vi "Replace Array Elements.vi"() -> ()   [LabVIEW 2019]
doc: "Demonstrates the use of the Replace Array Subset function."
panel:
  out "Case 4 - Replace One Column in 2D Array":dbl[][](array[numeric])
  out "Case 3 - Replace One Row in 2D Array":dbl[][](array[numeric])
  in  "Column Index":i32
  in  "Row Index":i32
  in  "Element Index":i32
  in  "New Element":dbl=9.99
  out "Case 2 - Replace One Element in 2D Array":dbl[][](array[numeric])
  out "Case 1 - Replace One Element in 1D Array":dbl[](array[numeric])
  in  "Original 2D Array":dbl[][](array[numeric])=[[0.0, 1.0, 2.0, 3.0], [4.0, 5.0, 6.0, 7.0], [8.0, 9.0, 10.0, 11.0], [12.0, 13.0, 14.0, 15.0]]
  in  "Original 1D Array":dbl[](array[numeric])=[100.0, 101.0, 102.0, 103.0]
  # "Overview: Demonstrates the use of the Replace Array Subset function.\nInstructions:\nRun the VI."
  # "Assign New Element into the 1D array at the position specified by Element Index."
  # "Assign New Element into the 2D array at the position specified by Row Index and Column Index."
  # "Assign Original 1D Array into the 2D array at the row specified by Row Index."
  # "Assign Original 1D Array into the 2D array at the column specified by Column Index."
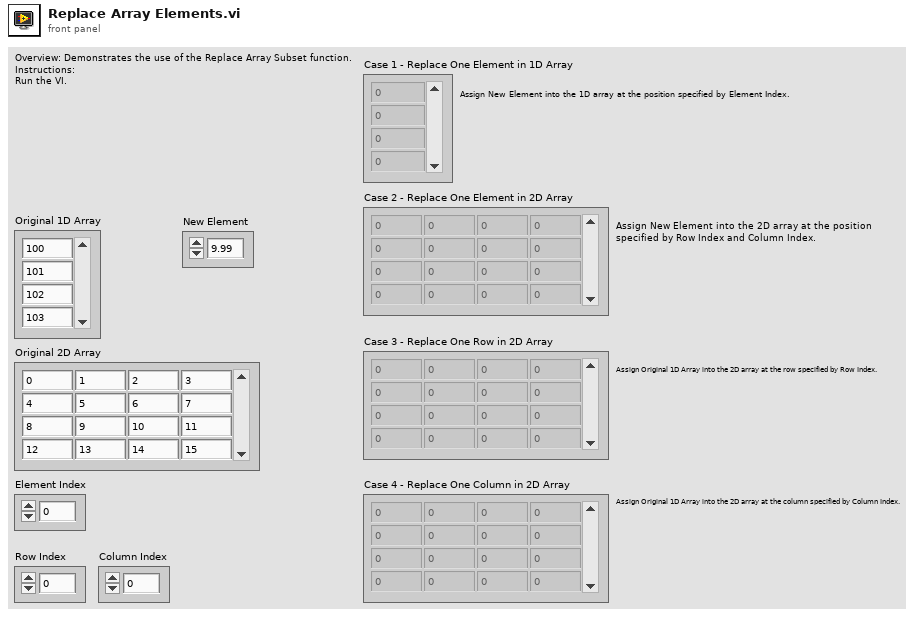
[diagram p1: front panel]
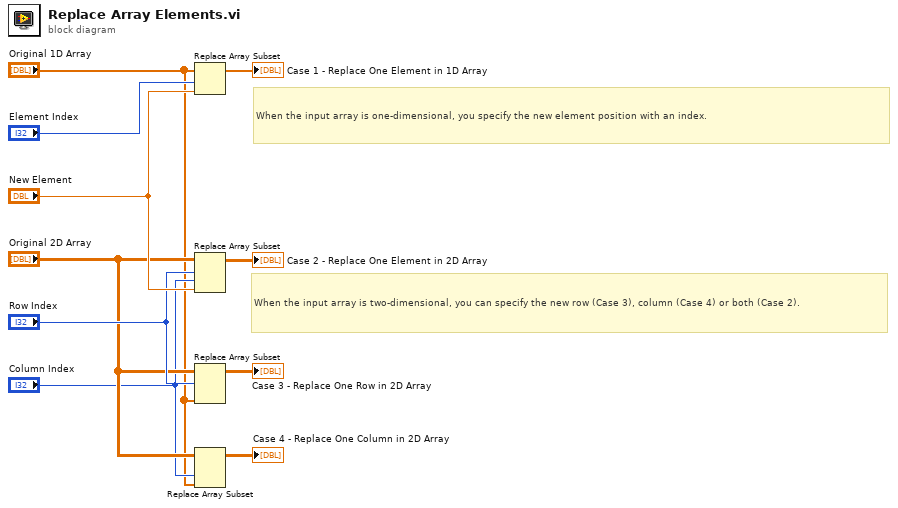
[diagram p0: block diagram]
diagram:
  # "When the input array is two-dimensional, you can specify the new row (Case 3), column (Case 4) or both (Case 2)."
  # "When the input array is one-dimensional, you specify the new element position with an index."
  n1 = Replace Array Subset(array="Original 1D Array", new element="New Element", index="Element Index") -> (→"Case 1 - Replace One Element in 1D Array":dbl[])
  n2 = Replace Array Subset(array="Original 2D Array", new element="New Element", index (row)="Row Index", index (col)="Column Index") -> (→"Case 2 - Replace One Element in 2D Array":dbl[][])
  n3 = Replace Array Subset(array="Original 2D Array", new element="Original 1D Array", index (row)="Row Index") -> (→"Case 3 - Replace One Row in 2D Array":dbl[][])  [unwired: 1 in]
  n4 = Replace Array Subset(array="Original 2D Array", new element="Original 1D Array", index (col)="Column Index") -> (→"Case 4 - Replace One Column in 2D Array":dbl[][])  [unwired: 1 in]
